vi "OE1022D_Read 1 parameter_mean.vi"(1 "数据转换":u8[](array[numeric]), 5 "Parameter 3":u16(ring) items=["AUX1", "AUX2", "AUX3", "AUX4"], 7 "Parameter 2":u16(ring) items=["X", "Y", "R", "Theta", "Frequency", "Noise", "Xh1", "Yh1", "Rh1", "Theta h1", "Xh2", "Yh2", "Rh2", "Theta h2"], 8 "错误输入（无错误）":errorcluster {"code" format="%f"}, 9 "Parameter":u16(ring) items=["X", "Y", "R", "Theta", "Frequency", "Noise", "Xh1", "Yh1", "Rh1", "Theta h1", "Xh2", "Yh2", "Rh2", "Theta h2"], 10 "Channel (0: A)":u16(ring) items=["Channel A", "Channel B", "ADC"], 11 "VISA resource name":refnum<visa-resource-name>) -> (0 "error out":errorcluster, 2 "Measurement":dbl format="%.3p", 3 "VISA resource name out":refnum<visa-resource-name>)   [LabVIEW 2024]
uses:
  <vilib>/Analysis/baseanly.llb/Mean (DBL).vi
  <vilib>/Analysis/NI_AALBase.lvlib
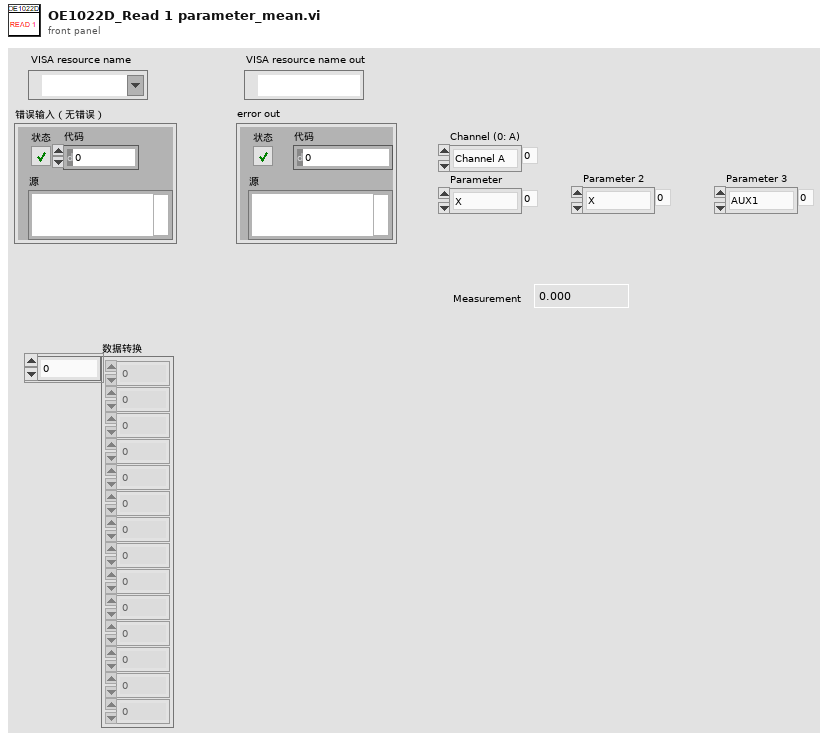
[diagram p1: front panel]
types:
  T1 = cluster{"AD1":dbl[], "AD2":dbl[], "AD3":dbl[], "AD4":dbl[]}
  T2 = cluster{"XA":dbl[], "YA":dbl[], "FrequencyA":dbl[], "NoiseA":dbl[], "Xh1A":dbl[], "Yh1A":dbl[], "Xh2A":dbl[], "Yh2A":dbl[]}
  T3 = cluster{"XB":dbl[], "YB":dbl[], "FrequencyB":dbl[], "NoiseB":dbl[], "Xh1B":dbl[], "Yh1B":dbl[], "Xh2B":dbl[], "Yh2B":dbl[], "Xh2B":dbl[]}
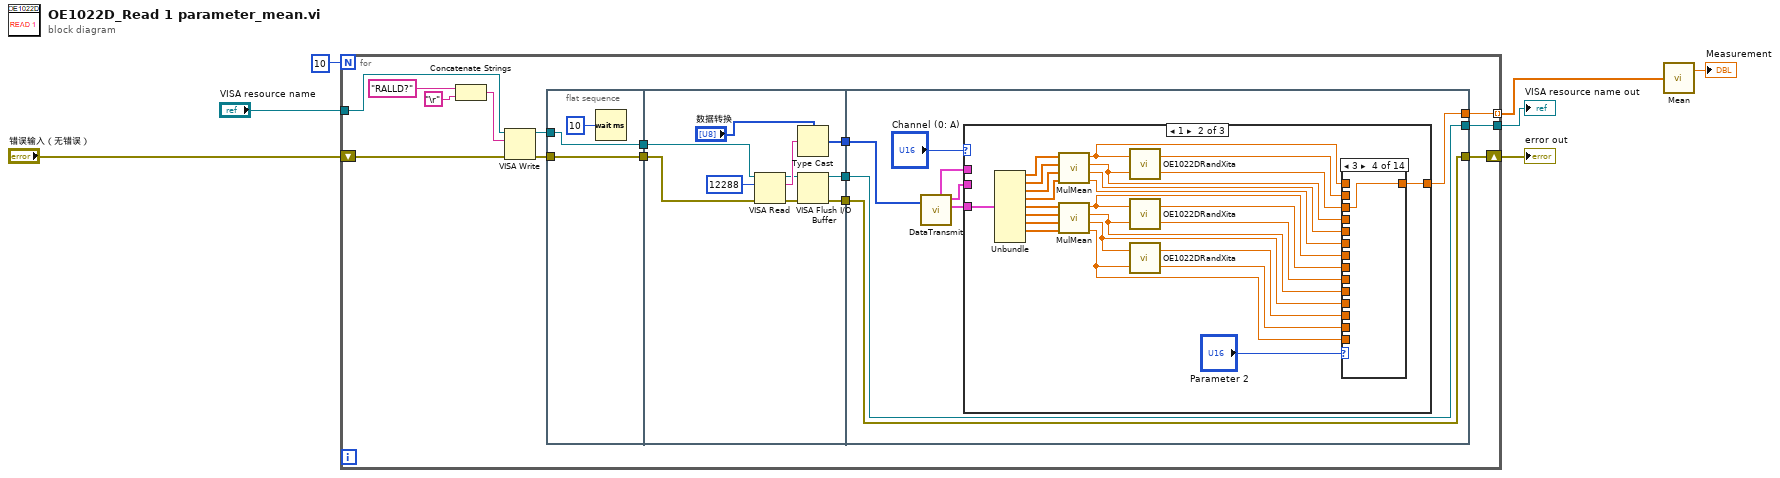
[diagram p0: block diagram]
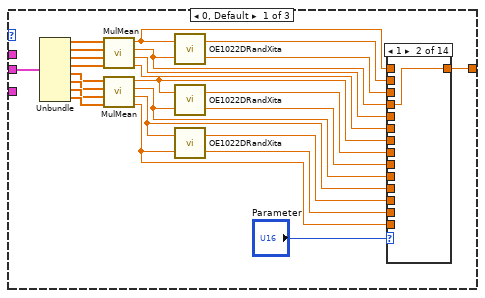
[diagram p2: hidden frame]
diagram:
  n1 = for {
    N: 10 -> [_]
    tunnel: [w12] -> w7
    shift-right: [w11] -> w6
    shift-left: "错误输入（无错误）" -> [w8]
    tunnel: [w10] -> w2 mode=indexing
    tunnel: "VISA resource name" -> [w9]
    n2 = Concatenate Strings("RALLD?" ("命令输入"), "\r") -> (w16:string)
    n3 = VISA Write(VISA resource name=w9, write buffer=w16, error in (no error)=w8) -> (VISA resource name out=w14:refnum<visa-resource-name>, error out=w13:errorcluster)  [unwired: 1 out]
    n4 = flat-sequence {
      tunnel: w14 -> [w23]
      tunnel: w13 -> [w24]
      tunnel: [w24] -> w22
      tunnel: [w23] -> w21
      tunnel: w22 -> [w27]
      tunnel: w21 -> [w26]
      tunnel: [w30] -> w20
      tunnel: [w29] -> w19
      tunnel: [w28] -> w18
      tunnel: w20 -> [w40]
      tunnel: w19 -> [w42]
      tunnel: w18 -> [w41]
      tunnel: [w42] -> w11
      tunnel: [w41] -> w12
      tunnel: [w36] -> w10
      frame #0 {
        n5 = Wait (ms)(milliseconds to wait=u32 10 ("等待时间（毫秒）")) -> ()  [unwired: 1 out]
      }
      frame #1 {
        n6 = VISA Read(VISA resource name=w26, byte count=12288, error in (no error)=w27) -> (VISA resource name out=w32:refnum<visa-resource-name>, read buffer=w34:string, error out=w33:errorcluster)  [unwired: 1 out]
        n7 = Type Cast(type="数据转换", x=w34) -> (*(type *) &x=w30:u8[])
        n8 = VISA Flush I/O Buffer(VISA resource name=w32, error in (no error)=w33) -> (VISA resource name out=w28:refnum<visa-resource-name>, error out=w29:errorcluster)  [unwired: 1 in]
      }
      frame #2 {
        n9 = call "DataTransmit.vi"("数据输入"=w40) -> ("输出簇ADC"=w39:T1, "输出簇A"=w38:T2, "输出簇B"=w37:T3)  [unwired: 2 in, 2 out]
        n10 = case shown="1" "Channel (0: A)" {
          tunnel: w39 -> [_ _ w128]
          tunnel: w38 -> [w59 _ _]
          tunnel: w37 -> [_ w83 _]
          tunnel: [w54 w84 w122] -> w36
          frame 0, Default {
            n11 = Unbundle(w59) -> ("XA"=w60:dbl[], "YA"=w61:dbl[], "FrequencyA"=w62:dbl[], "NoiseA"=w63:dbl[], "Xh1A"=w64:dbl[], "Yh1A"=w65:dbl[], "Xh2A"=w66:dbl[], "Yh2A"=w67:dbl[])
            n12 = call "MulMean.vi"("IN 4"=w63, "IN 3"=w62, "IN 2"=w61, "IN 1"=w60) -> ("mean 4"=w48:dbl, "mean 3"=w49:dbl, "mean 2"=w57:dbl, "mean 1"=w58:dbl)  [unwired: 4 in]
            n13 = call "MulMean.vi"("IN 4"=w67, "IN 3"=w66, "IN 2"=w65, "IN 1"=w64) -> ("mean 4"=w46:dbl, "mean 3"=w47:dbl, "mean 2"=w52:dbl, "mean 1"=w53:dbl)  [unwired: 4 in]
            n14 = call "OE1022DRandXita.vi"("Y"=w57, "X"=w58) -> ("θ (°)"=w55:dbl, "R"=w56:dbl)
            n15 = call "OE1022DRandXita.vi"("Y"=w52, "X"=w53) -> ("θ (°)"=w50:dbl, "R"=w51:dbl)
            n16 = call "OE1022DRandXita.vi"("Y"=w46, "X"=w47) -> ("θ (°)"=w44:dbl, "R"=w45:dbl)
            n17 = case shown="1" "Parameter" {
              tunnel: w58 -> [w69 _ _ _ _ _ _ _ _ _ _ _ _ _]
              tunnel: w57 -> [_ w70 _ _ _ _ _ _ _ _ _ _ _ _]
              tunnel: w56 -> [_ _ w71 _ _ _ _ _ _ _ _ _ _ _]
              tunnel: w55 -> [_ _ _ w72 _ _ _ _ _ _ _ _ _ _]
              tunnel: [w69 w70 w71 w72 w73 w74 w75 w76 w77 w78 w79 w80 w81 w82] -> w54
              tunnel: w53 -> [_ _ _ _ _ _ w75 _ _ _ _ _ _ _]
              tunnel: w52 -> [_ _ _ _ _ _ _ w76 _ _ _ _ _ _]
              tunnel: w51 -> [_ _ _ _ _ _ _ _ w77 _ _ _ _ _]
              tunnel: w50 -> [_ _ _ _ _ _ _ _ _ w78 _ _ _ _]
              tunnel: w49 -> [_ _ _ _ w73 _ _ _ _ _ _ _ _ _]
              tunnel: w48 -> [_ _ _ _ _ w74 _ _ _ _ _ _ _ _]
              tunnel: w47 -> [_ _ _ _ _ _ _ _ _ _ w79 _ _ _]
              tunnel: w46 -> [_ _ _ _ _ _ _ _ _ _ _ w80 _ _]
              tunnel: w45 -> [_ _ _ _ _ _ _ _ _ _ _ _ w81 _]
              tunnel: w44 -> [_ _ _ _ _ _ _ _ _ _ _ _ _ w82]
              frame 0, Default {
              }
              frame 1 {
              }
              frame 2 {
              }
              frame 3 {
              }
              frame 4 {
              }
              frame 5 {
              }
              frame 6 {
              }
              frame 7 {
              }
              frame 8 {
              }
              frame 9 {
              }
              frame 10 {
              }
              frame 11 {
              }
              frame 12 {
              }
              frame 13 {
              }
            }
          }
          frame 1 {
            n18 = Unbundle(w83) -> ("XB"=w93:dbl[], "YB"=w92:dbl[], "FrequencyB"=w91:dbl[], "NoiseB"=w90:dbl[], "Xh1B"=w89:dbl[], "Yh1B"=w88:dbl[], "Xh2B"=w87:dbl[], "Yh2B"=w86:dbl[])  [unwired: 1 out]
            n19 = call "MulMean.vi"("IN 4"=w90, "IN 3"=w91, "IN 2"=w92, "IN 1"=w93) -> ("mean 4"=w103:dbl, "mean 3"=w102:dbl, "mean 2"=w95:dbl, "mean 1"=w94:dbl)  [unwired: 4 in]
            n20 = call "MulMean.vi"("IN 4"=w86, "IN 3"=w87, "IN 2"=w88, "IN 1"=w89) -> ("mean 4"=w105:dbl, "mean 3"=w104:dbl, "mean 2"=w99:dbl, "mean 1"=w98:dbl)  [unwired: 4 in]
            n21 = call "OE1022DRandXita.vi"("Y"=w95, "X"=w94) -> ("θ (°)"=w97:dbl, "R"=w96:dbl)
            n22 = call "OE1022DRandXita.vi"("Y"=w99, "X"=w98) -> ("θ (°)"=w101:dbl, "R"=w100:dbl)
            n23 = call "OE1022DRandXita.vi"("Y"=w105, "X"=w104) -> ("θ (°)"=w107:dbl, "R"=w106:dbl)
            n24 = case shown="3" "Parameter 2" {
              tunnel: w94 -> [w108 _ _ _ _ _ _ _ _ _ _ _ _ _]
              tunnel: w95 -> [_ w109 _ _ _ _ _ _ _ _ _ _ _ _]
              tunnel: w96 -> [_ _ w110 _ _ _ _ _ _ _ _ _ _ _]
              tunnel: w97 -> [_ _ _ w111 _ _ _ _ _ _ _ _ _ _]
              tunnel: [w108 w109 w110 w111 w112 w113 w114 w115 w116 w117 w118 w119 w120 w121] -> w84
              tunnel: w98 -> [_ _ _ _ _ _ w114 _ _ _ _ _ _ _]
              tunnel: w99 -> [_ _ _ _ _ _ _ w115 _ _ _ _ _ _]
              tunnel: w100 -> [_ _ _ _ _ _ _ _ w116 _ _ _ _ _]
              tunnel: w101 -> [_ _ _ _ _ _ _ _ _ w117 _ _ _ _]
              tunnel: w102 -> [_ _ _ _ w112 _ _ _ _ _ _ _ _ _]
              tunnel: w103 -> [_ _ _ _ _ w113 _ _ _ _ _ _ _ _]
              tunnel: w104 -> [_ _ _ _ _ _ _ _ _ _ w118 _ _ _]
              tunnel: w105 -> [_ _ _ _ _ _ _ _ _ _ _ w119 _ _]
              tunnel: w106 -> [_ _ _ _ _ _ _ _ _ _ _ _ w120 _]
              tunnel: w107 -> [_ _ _ _ _ _ _ _ _ _ _ _ _ w121]
              frame 0, Default {
              }
              frame 1 {
              }
              frame 2 {
              }
              frame 3 {
              }
              frame 4 {
              }
              frame 5 {
              }
              frame 6 {
              }
              frame 7 {
              }
              frame 8 {
              }
              frame 9 {
              }
              frame 10 {
              }
              frame 11 {
              }
              frame 12 {
              }
              frame 13 {
              }
            }
          }
          frame 2 {
            n25 = Unbundle By Name(w128) -> ("AD1"=w132:dbl[], "AD2"=w131:dbl[], "AD3"=w130:dbl[], "AD4"=w129:dbl[])
            n26 = call "MulMean.vi"("IN 4"=w129, "IN 3"=w130, "IN 2"=w131, "IN 1"=w132) -> ("mean 4"=w123:dbl, "mean 3"=w124:dbl, "mean 2"=w125:dbl, "mean 1"=w126:dbl)  [unwired: 4 in]
            n27 = case shown="3" "Parameter 3" {
              tunnel: w126 -> [w133 _ _ _]
              tunnel: w125 -> [_ w134 _ _]
              tunnel: w124 -> [_ _ w135 _]
              tunnel: w123 -> [_ _ _ w136]
              tunnel: [w133 w134 w135 w136] -> w122
              frame 0, Default {
              }
              frame 1 {
              }
              frame 2 {
              }
              frame 3 {
              }
            }
          }
        }
      }
    }
  }
  "VISA resource name out" <- w7
  "error out" <- w6
  n28 = call-poly <vilib>:"Mean.vi"("X"=w2) -> ("mean"=→"Measurement":dbl)  [unwired: 1 out]
